vi "IV(H)_DC_vector_magnet_anglesweep_BF_LD-400_K6221_K2182A_PK.vi"() -> ()   [LabVIEW 2016]
uses:
  <vilib>/Math Plots/2D Math Plots/2D Compass/2D Compass XCtrl/2D Compass.xctl
  <vilib>/Math Plots/2D Math Plots/2D Compass/2D Compass Datatype/2D Compass Datatype.lvclass
  <vilib>/Math Plots/2D Math Plots/2D Compass/2D Compass Datatype/Public/Plot Helper (Vector).vi
  Labview Drivers/Keithley 622x LV 2009/Keithley 622x.lvlib
panel:
  out "2D Compass":refnum<class "2D Plot Datatype.lvclass">[](xcontrol)
  in  "Set Compliance voltage (V)":dbl=5.0 min=0.0 step=0.1 format="%_3f"
  in  "Step 3":dbl[](array[numeric])=[2e-06, 0.0001, 2e-06, 1e-06] min=-3000.0 max=3000.0 format="%.3e"
  in  "To 3":dbl[](array[numeric])=[0.00032, 1e-06, -0.00032, -1e-06] min=-3000.0 max=3000.0 format="%.1e"
  in  "From 3":dbl[](array[numeric])=[0.0, 0.00032, 0.0, -0.00032] min=-3000.0 max=3000.0 format="%.1e"
  in  "wait (ms)":u32=50
  in  "Nanovoltmeter 2182a VISA":refnum<visa-resource-name>="GPIB0::7::INSTR"
  in  "Current source K6221 VISA":refnum<visa-resource-name>="GPIB0::13::INSTR"
  in  "Number Averaging":i32=1
  in  "Tab Control":enum32{"Page 1", "Page 2"}(tab)
  out "V vs I":cluster{dbl, "Field Reading":dbl}[](graph)=[{0.0, "Field Reading"=4.40241798e-08}, {2e-08, "Field Reading"=1.23783257e-07}, {4e-08, "Field Reading"=3.02986118e-07}, {6e-08, "Field Reading"=5.49519534e-07}, {8e-08, "Field Reading"=7.0386157e-07}, {1e-07, "Field Reading"=8.50435e-07}, {1.2e-07, "Field Reading"=1.09593255e-06}, {1.4e-07, "Field Reading"=1.21350074e-06}, {1.6e-07, "Field Reading"=1.39529319e-06}, {1.8e-07, "Field Reading"=1.54134866e-06}, {2e-07, "Field Reading"=1.75991058e-06}, {2.2e-07, "Field Reading"=1.91891414e-06}, {2.4e-07, "Field Reading"=2.05875441e-06}, {2.6e-07, "Field Reading"=2.23173979e-06}, {2.8e-07, "Field Reading"=2.36018563e-06}, {3e-07, "Field Reading"=2.64452742e-06}, {3.2e-07, "Field Reading"=2.75122088e-06}, {3.4e-07, "Field Reading"=2.90763477e-06}, {3.6e-07, "Field Reading"=3.12050268e-06}, {3.8e-07, "Field Reading"=3.23392292e-06}, {4e-07, "Field Reading"=3.48200967e-06}, {4.2e-07, "Field Reading"=3.63013662e-06}, {4.4e-07, "Field Reading"=3.79483537e-06}, {4.6e-07, "Field Reading"=3.94296229e-06}, {4.8e-07, "Field Reading"=4.10869871e-06}, {5e-07, "Field Reading"=4.332443e-06}, {5.2e-07, "Field Reading"=4.44638679e-06}, {5.4e-07, "Field Reading"=4.61160528e-06}, {5.6e-07, "Field Reading"=4.8415635e-06}, {5.8e-07, "Field Reading"=4.99228004e-06}, {6e-07, "Field Reading"=5.17562593e-06}, {6.2e-07, "Field Reading"=5.33774246e-06}, {6.4e-07, "Field Reading"=5.53403662e-06}, {6.6e-07, "Field Reading"=5.65315972e-06}, {6.8e-07, "Field Reading"=5.83340484e-06}, {7e-07, "Field Reading"=6.04161144e-06}, {7.2e-07, "Field Reading"=6.14312511e-06}, {7.4e-07, "Field Reading"=6.37827086e-06}, {7.6e-07, "Field Reading"=6.53727451e-06}, {7.8e-07, "Field Reading"=6.69938572e-06}, {8e-07, "Field Reading"=6.88635475e-06}, {8.2e-07, "Field Reading"=7.02101579e-06}, {8.4e-07, "Field Reading"=7.23699138e-06}, {8.6e-07, "Field Reading"=7.41308471e-06}, {8.8e-07, "Field Reading"=7.58244684e-06}, {9e-07, "Field Reading"=7.74041457e-06}, {9.2e-07, "Field Reading"=7.90562381e-06}, {9.4e-07, "Field Reading"=8.06618106e-06}, {9.6e-07, "Field Reading"=8.2422761e-06}, {9.8e-07, "Field Reading"=8.41162272e-06}, {1e-06, "Field Reading"=8.59082511e-06}, {1.02e-06, "Field Reading"=8.73842623e-06}, {1.04e-06, "Field Reading"=8.94248895e-06}, {1.06e-06, "Field Reading"=9.14240827e-06}, {1.08e-06, "Field Reading"=9.27862314e-06}, {1.1e-06, "Field Reading"=9.47388113e-06}, {1.12e-06, "Field Reading"=9.62770506e-06}, {1.14e-06, "Field Reading"=9.81261485e-06}, {1.16e-06, "Field Reading"=9.94365015e-06}, {1.18e-06, "Field Reading"=1.0168948e-05}, {1.2e-06, "Field Reading"=1.03238199e-05}, {1.22e-06, "Field Reading"=1.05263292e-05}, {1.24e-06, "Field Reading"=1.0654257e-05}, {1.26e-06, "Field Reading"=1.08365675e-05}, {1.28e-06, "Field Reading"=1.09608698e-05}, {1.3e-06, "Field Reading"=1.11291959e-05}, {1.32e-06, "Field Reading"=1.13104759e-05}, {1.34e-06, "Field Reading"=1.14658539e-05}, {1.36e-06, "Field Reading"=1.17056539e-05}, {1.38e-06, "Field Reading"=1.1880715e-05}, {1.4e-06, "Field Reading"=1.20252166e-05}, {1.42e-06, "Field Reading"=1.22121882e-05}, {1.44e-06, "Field Reading"=1.23541037e-05}, {1.46e-06, "Field Reading"=1.2493426e-05}, {1.48e-06, "Field Reading"=1.27368517e-05}, {1.5e-06, "Field Reading"=1.28668613e-05}, {1.52e-06, "Field Reading"=1.3010845e-05}, {1.54e-06, "Field Reading"=1.31729562e-05}, {1.56e-06, "Field Reading"=1.34153398e-05}, {1.58e-06, "Field Reading"=1.3541714e-05}, {1.6e-06, "Field Reading"=1.36877694e-05}, {1.62e-06, "Field Reading"=1.38659327e-05}, {1.64e-06, "Field Reading"=1.40705138e-05}, {1.66e-06, "Field Reading"=1.42554137e-05}, {1.68e-06, "Field Reading"=1.43978348e-05}, {1.7e-06, "Field Reading"=1.45537307e-05}, {1.72e-06, "Field Reading"=1.4763491e-05}, {1.74e-06, "Field Reading"=1.49478731e-05}, {1.76e-06, "Field Reading"=1.50571556e-05}, {1.78e-06, "Field Reading"=1.5244645e-05}, {1.8e-06, "Field Reading"=1.54171202e-05}, {1.82e-06, "Field Reading"=1.55590321e-05}, {1.84e-06, "Field Reading"=1.57708642e-05}, {1.86e-06, "Field Reading"=1.59593796e-05}, {1.88e-06, "Field Reading"=1.60826461e-05}, {1.9e-06, "Field Reading"=1.62836016e-05}, {1.92e-06, "Field Reading"=1.64534904e-05}, {1.94e-06, "Field Reading"=1.65871155e-05}, {1.96e-06, "Field Reading"=1.68072344e-05}, {1.98e-06, "Field Reading"=1.69807332e-05}, {2e-06, "Field Reading"=1.71039997e-05}, {2.02e-06, "Field Reading"=1.73298157e-05}, {2.04e-06, "Field Reading"=1.75338777e-05}, {2.06e-06, "Field Reading"=1.76706104e-05}, {2.08e-06, "Field Reading"=1.78063071e-05}, {2.1e-06, "Field Reading"=1.79881126e-05}, {2.12e-06, "Field Reading"=1.81730125e-05}, {2.14e-06, "Field Reading"=1.83542869e-05}, {2.16e-06, "Field Reading"=1.84765118e-05}, {2.18e-06, "Field Reading"=1.86950769e-05}, {2.2e-06, "Field Reading"=1.88804946e-05}, {2.22e-06, "Field Reading"=1.90384784e-05}, {2.24e-06, "Field Reading"=1.91767649e-05}, {2.26e-06, "Field Reading"=1.93580394e-05}, {2.28e-06, "Field Reading"=1.95553725e-05}, {2.3e-06, "Field Reading"=1.97330215e-05}, {2.32e-06, "Field Reading"=1.98827024e-05}, {2.34e-06, "Field Reading"=2.00670785e-05}, {2.36e-06, "Field Reading"=2.02561219e-05}, {2.38e-06, "Field Reading"=2.04550059e-05}, {2.4e-06, "Field Reading"=2.05839566e-05}, {2.42e-06, "Field Reading"=2.07004901e-05}, {2.44e-06, "Field Reading"=2.08941947e-05}, {2.46e-06, "Field Reading"=2.10935914e-05}, {2.48e-06, "Field Reading"=2.12541486e-05}, {2.5e-06, "Field Reading"=2.14209052e-05}, {2.52e-06, "Field Reading"=2.16146097e-05}, {2.54e-06, "Field Reading"=2.18026169e-05}, {2.56e-06, "Field Reading"=2.19916641e-05}, {2.58e-06, "Field Reading"=2.21568827e-05}, {2.6e-06, "Field Reading"=2.23319418e-05}, {2.62e-06, "Field Reading"=2.2459882e-05}, {2.64e-06, "Field Reading"=2.26406384e-05}, {2.66e-06, "Field Reading"=2.28395223e-05}, {2.68e-06, "Field Reading"=2.2994903e-05}, {2.7e-06, "Field Reading"=2.31471734e-05}, {2.72e-06, "Field Reading"=2.32978901e-05}, {2.74e-06, "Field Reading"=2.34921259e-05}, {2.76e-06, "Field Reading"=2.36547549e-05}, {2.78e-06, "Field Reading"=2.38215274e-05}, {2.8e-06, "Field Reading"=2.40152458e-05}, {2.82e-06, "Field Reading"=2.41934127e-05}, {2.84e-06, "Field Reading"=2.43938505e-05}, {2.86e-06, "Field Reading"=2.4514533e-05}, {2.88e-06, "Field Reading"=2.47548513e-05}, {2.9e-06, "Field Reading"=2.48532575e-05}, {2.92e-06, "Field Reading"=2.50619679e-05}, {2.94e-06, "Field Reading"=2.51930034e-05}, {2.96e-06, "Field Reading"=2.5380493e-05}, {2.98e-06, "Field Reading"=2.55322419e-05}, {3e-06, "Field Reading"=2.57492533e-05}, {3e-06, "Field Reading"=2.57720421e-05}, {2e-06, "Field Reading"=1.71412944e-05}, {1e-06, "Field Reading"=8.50279535e-06}, {0.0, "Field Reading"=-1.17576765e-07}, {-2e-08, "Field Reading"=-2.68811351e-07}, {-4e-08, "Field Reading"=-4.69766897e-07}, {-6e-08, "Field Reading"=-6.21518846e-07}, {-8e-08, "Field Reading"=-8.17295154e-07}, {-1e-07, "Field Reading"=-9.41079645e-07}, {-1.2e-07, "Field Reading"=-1.18502315e-06}, {-1.4e-07, "Field Reading"=-1.34454459e-06}, {-1.6e-07, "Field Reading"=-1.46573945e-06}, {-1.8e-07, "Field Reading"=-1.69051911e-06}, {-2e-07, "Field Reading"=-1.82621594e-06}, {-2.2e-07, "Field Reading"=-2.0126696e-06}, {-2.4e-07, "Field Reading"=-2.21776914e-06}, {-2.6e-07, "Field Reading"=-2.35450179e-06}, {-2.8e-07, "Field Reading"=-2.58601504e-06}, {-3e-07, "Field Reading"=-2.69322674e-06}, {-3.2e-07, "Field Reading"=-2.83721031e-06}, {-3.4e-07, "Field Reading"=-3.08995843e-06}, {-3.6e-07, "Field Reading"=-3.19457944e-06}, {-3.8e-07, "Field Reading"=-3.37844337e-06}, {-4e-07, "Field Reading"=-3.57266625e-06}, {-4.2e-07, "Field Reading"=-3.76792448e-06}, {-4.4e-07, "Field Reading"=-3.93469675e-06}, {-4.6e-07, "Field Reading"=-4.04864062e-06}, {-4.8e-07, "Field Reading"=-4.20505435e-06}, {-5e-07, "Field Reading"=-4.46867881e-06}, {-5.2e-07, "Field Reading"=-4.63596869e-06}, {-5.4e-07, "Field Reading"=-4.79238132e-06}, {-5.6e-07, "Field Reading"=-4.99799659e-06}, {-5.8e-07, "Field Reading"=-5.13783554e-06}, {-6e-07, "Field Reading"=-5.31133956e-06}, {-6.2e-07, "Field Reading"=-5.45014278e-06}, {-6.4e-07, "Field Reading"=-5.69460221e-06}, {-6.6e-07, "Field Reading"=-5.77436228e-06}, {-6.8e-07, "Field Reading"=-5.97428035e-06}, {-7e-07, "Field Reading"=-6.12913905e-06}, {-7.2e-07, "Field Reading"=-6.38136727e-06}, {-7.4e-07, "Field Reading"=-6.52534971e-06}, {-7.6e-07, "Field Reading"=-6.63359599e-06}, {-7.8e-07, "Field Reading"=-6.85112346e-06}, {-8e-07, "Field Reading"=-7.07020515e-06}, {-8.2e-07, "Field Reading"=-7.20641881e-06}, {-8.4e-07, "Field Reading"=-7.40167564e-06}, {-8.6e-07, "Field Reading"=-7.54669386e-06}, {-8.8e-07, "Field Reading"=-7.71035741e-06}, {-9e-07, "Field Reading"=-7.89525579e-06}, {-9.2e-07, "Field Reading"=-8.04286623e-06}, {-9.4e-07, "Field Reading"=-8.20031482e-06}, {-9.6e-07, "Field Reading"=-8.37226526e-06}, {-9.8e-07, "Field Reading"=-8.56441587e-06}, {-1e-06, "Field Reading"=-8.75760121e-06}, {-1.02e-06, "Field Reading"=-8.97305724e-06}, {-1.04e-06, "Field Reading"=-9.09994792e-06}, {-1.06e-06, "Field Reading"=-9.267755e-06}, {-1.08e-06, "Field Reading"=-9.48372893e-06}, {-1.1e-06, "Field Reading"=-9.64739249e-06}, {-1.12e-06, "Field Reading"=-9.79396472e-06}, {-1.14e-06, "Field Reading"=-9.97938118e-06}, {-1.16e-06, "Field Reading"=-1.00990192e-05}, {-1.18e-06, "Field Reading"=-1.03647137e-05}, {-1.2e-06, "Field Reading"=-1.04952302e-05}, {-1.22e-06, "Field Reading"=-1.06247112e-05}, {-1.24e-06, "Field Reading"=-1.08479359e-05}, {-1.26e-06, "Field Reading"=-1.10452646e-05}, {-1.28e-06, "Field Reading"=-1.11291712e-05}, {-1.3e-06, "Field Reading"=-1.13979733e-05}, {-1.32e-06, "Field Reading"=-1.15290079e-05}, {-1.34e-06, "Field Reading"=-1.17107996e-05}, {-1.36e-06, "Field Reading"=-1.18584077e-05}, {-1.38e-06, "Field Reading"=-1.2031394e-05}, {-1.4e-06, "Field Reading"=-1.22214705e-05}, {-1.42e-06, "Field Reading"=-1.23742578e-05}, {-1.44e-06, "Field Reading"=-1.25384394e-05}, {-1.46e-06, "Field Reading"=-1.27621798e-05}, {-1.48e-06, "Field Reading"=-1.28792304e-05}, {-1.5e-06, "Field Reading"=-1.30289101e-05}, {-1.52e-06, "Field Reading"=-1.32428105e-05}, {-1.54e-06, "Field Reading"=-1.34660352e-05}, {-1.56e-06, "Field Reading"=-1.35644406e-05}, {-1.58e-06, "Field Reading"=-1.37255157e-05}, {-1.6e-06, "Field Reading"=-1.39409717e-05}, {-1.62e-06, "Field Reading"=-1.41439974e-05}, {-1.64e-06, "Field Reading"=-1.42952297e-05}, {-1.66e-06, "Field Reading"=-1.44941121e-05}, {-1.68e-06, "Field Reading"=-1.45919995e-05}, {-1.7e-06, "Field Reading"=-1.47965808e-05}, {-1.72e-06, "Field Reading"=-1.50275744e-05}, {-1.74e-06, "Field Reading"=-1.51088883e-05}, {-1.76e-06, "Field Reading"=-1.5286534e-05}, {-1.78e-06, "Field Reading"=-1.55475671e-05}, {-1.8e-06, "Field Reading"=-1.56418291e-05}, {-1.82e-06, "Field Reading"=-1.58401957e-05}, {-1.84e-06, "Field Reading"=-1.60354527e-05}, {-1.86e-06, "Field Reading"=-1.61778815e-05}, {-1.88e-06, "Field Reading"=-1.64109433e-05}, {-1.9e-06, "Field Reading"=-1.65114203e-05}, {-1.92e-06, "Field Reading"=-1.67460393e-05}, {-1.94e-06, "Field Reading"=-1.69164354e-05}, {-1.96e-06, "Field Reading"=-1.7107031e-05}, {-1.98e-06, "Field Reading"=-1.72157948e-05}, {-2e-06, "Field Reading"=-1.73789424e-05}, {-2.02e-06, "Field Reading"=-1.7616151e-05}, {-2.04e-06, "Field Reading"=-1.77135205e-05}, {-2.06e-06, "Field Reading"=-1.788599e-05}, {-2.08e-06, "Field Reading"=-1.80781394e-05}, {-2.1e-06, "Field Reading"=-1.82045126e-05}, {-2.12e-06, "Field Reading"=-1.84603712e-05}, {-2.14e-06, "Field Reading"=-1.8589852e-05}, {-2.16e-06, "Field Reading"=-1.87690534e-05}, {-2.18e-06, "Field Reading"=-1.89917572e-05}, {-2.2e-06, "Field Reading"=-1.91388473e-05}, {-2.22e-06, "Field Reading"=-1.93584466e-05}, {-2.24e-06, "Field Reading"=-1.95366097e-05}, {-2.26e-06, "Field Reading"=-1.96655725e-05}, {-2.28e-06, "Field Reading"=-1.98468455e-05}, {-2.3e-06, "Field Reading"=-2.00260392e-05}, {-2.32e-06, "Field Reading"=-2.02104196e-05}, {-2.34e-06, "Field Reading"=-2.03642427e-05}, {-2.36e-06, "Field Reading"=-2.05486354e-05}, {-2.38e-06, "Field Reading"=-2.07009048e-05}, {-2.4e-06, "Field Reading"=-2.08485128e-05}, {-2.42e-06, "Field Reading"=-2.10551707e-05}, {-2.44e-06, "Field Reading"=-2.12468023e-05}, {-2.46e-06, "Field Reading"=-2.14161632e-05}, {-2.48e-06, "Field Reading"=-2.1574128e-05}, {-2.5e-06, "Field Reading"=-2.17181107e-05}, {-2.52e-06, "Field Reading"=-2.18755593e-05}, {-2.54e-06, "Field Reading"=-2.21179489e-05}, {-2.56e-06, "Field Reading"=-2.22878278e-05}, {-2.58e-06, "Field Reading"=-2.246185e-05}, {-2.6e-06, "Field Reading"=-2.26146323e-05}, {-2.62e-06, "Field Reading"=-2.28161044e-05}, {-2.64e-06, "Field Reading"=-2.29424776e-05}, {-2.66e-06, "Field Reading"=-2.30880191e-05}, {-2.68e-06, "Field Reading"=-2.32863837e-05}, {-2.7e-06, "Field Reading"=-2.34681748e-05}, {-2.72e-06, "Field Reading"=-2.36484132e-05}, {-2.74e-06, "Field Reading"=-2.38566183e-05}, {-2.76e-06, "Field Reading"=-2.39985293e-05}, {-2.78e-06, "Field Reading"=-2.41513117e-05}, {-2.8e-06, "Field Reading"=-2.43227442e-05}, {-2.82e-06, "Field Reading"=-2.44646552e-05}, {-2.84e-06, "Field Reading"=-2.46112313e-05}, {-2.86e-06, "Field Reading"=-2.47919865e-05}, {-2.88e-06, "Field Reading"=-2.50271236e-05}, {-2.9e-06, "Field Reading"=-2.51327718e-05}, {-2.92e-06, "Field Reading"=-2.53295825e-05}, {-2.94e-06, "Field Reading"=-2.55269109e-05}, {-2.96e-06, "Field Reading"=-2.57024868e-05}, {-2.98e-06, "Field Reading"=-2.5883242e-05}, {-3e-06, "Field Reading"=-2.59930485e-05}, {-3e-06, "Field Reading"=-2.60981869e-05}, {-2e-06, "Field Reading"=-1.74783916e-05}]
  out "V vs time":cluster{dbl, "Field Reading":dbl}[](graph)=[{14037.38, "Field Reading"=4.40241798e-08}, {14037.632, "Field Reading"=1.23783257e-07}, {14037.885, "Field Reading"=3.02986118e-07}, {14038.144, "Field Reading"=5.49519534e-07}, {14038.396, "Field Reading"=7.0386157e-07}, {14038.649, "Field Reading"=8.50435e-07}, {14038.901, "Field Reading"=1.09593255e-06}, {14039.16, "Field Reading"=1.21350074e-06}, {14039.412, "Field Reading"=1.39529319e-06}, {14039.666, "Field Reading"=1.54134866e-06}, {14039.921, "Field Reading"=1.75991058e-06}, {14040.178, "Field Reading"=1.91891414e-06}, {14040.432, "Field Reading"=2.05875441e-06}, {14040.684, "Field Reading"=2.23173979e-06}, {14040.944, "Field Reading"=2.36018563e-06}, {14041.201, "Field Reading"=2.64452742e-06}, {14041.453, "Field Reading"=2.75122088e-06}, {14041.705, "Field Reading"=2.90763477e-06}, {14041.964, "Field Reading"=3.12050268e-06}, {14042.218, "Field Reading"=3.23392292e-06}, {14042.47, "Field Reading"=3.48200967e-06}, {14042.726, "Field Reading"=3.63013662e-06}, {14042.982, "Field Reading"=3.79483537e-06}, {14043.242, "Field Reading"=3.94296229e-06}, {14043.495, "Field Reading"=4.10869871e-06}, {14043.747, "Field Reading"=4.332443e-06}, {14043.999, "Field Reading"=4.44638679e-06}, {14044.252, "Field Reading"=4.61160528e-06}, {14044.507, "Field Reading"=4.8415635e-06}, {14044.761, "Field Reading"=4.99228004e-06}, {14045.019, "Field Reading"=5.17562593e-06}, {14045.274, "Field Reading"=5.33774246e-06}, {14045.526, "Field Reading"=5.53403662e-06}, {14045.778, "Field Reading"=5.65315972e-06}, {14046.028, "Field Reading"=5.83340484e-06}, {14046.282, "Field Reading"=6.04161144e-06}, {14046.538, "Field Reading"=6.14312511e-06}, {14046.794, "Field Reading"=6.37827086e-06}, {14047.048, "Field Reading"=6.53727451e-06}, {14047.299, "Field Reading"=6.69938572e-06}, {14047.553, "Field Reading"=6.88635475e-06}, {14047.806, "Field Reading"=7.02101579e-06}, {14048.061, "Field Reading"=7.23699138e-06}, {14048.315, "Field Reading"=7.41308471e-06}, {14048.572, "Field Reading"=7.58244684e-06}, {14048.825, "Field Reading"=7.74041457e-06}, {14049.076, "Field Reading"=7.90562381e-06}, {14049.332, "Field Reading"=8.06618106e-06}, {14049.585, "Field Reading"=8.2422761e-06}, {14049.845, "Field Reading"=8.41162272e-06}, {14050.098, "Field Reading"=8.59082511e-06}, {14050.354, "Field Reading"=8.73842623e-06}, {14050.61, "Field Reading"=8.94248895e-06}, {14050.867, "Field Reading"=9.14240827e-06}, {14051.121, "Field Reading"=9.27862314e-06}, {14051.375, "Field Reading"=9.47388113e-06}, {14051.632, "Field Reading"=9.62770506e-06}, {14051.888, "Field Reading"=9.81261485e-06}, {14052.138, "Field Reading"=9.94365015e-06}, {14052.392, "Field Reading"=1.0168948e-05}, {14052.645, "Field Reading"=1.03238199e-05}, {14052.897, "Field Reading"=1.05263292e-05}, {14053.15, "Field Reading"=1.0654257e-05}, {14053.405, "Field Reading"=1.08365675e-05}, {14053.659, "Field Reading"=1.09608698e-05}, {14053.913, "Field Reading"=1.11291959e-05}, {14054.167, "Field Reading"=1.13104759e-05}, {14054.419, "Field Reading"=1.14658539e-05}, {14054.67, "Field Reading"=1.17056539e-05}, {14054.922, "Field Reading"=1.1880715e-05}, {14055.177, "Field Reading"=1.20252166e-05}, {14055.434, "Field Reading"=1.22121882e-05}, {14055.689, "Field Reading"=1.23541037e-05}, {14055.94, "Field Reading"=1.2493426e-05}, {14056.191, "Field Reading"=1.27368517e-05}, {14056.449, "Field Reading"=1.28668613e-05}, {14056.699, "Field Reading"=1.3010845e-05}, {14056.952, "Field Reading"=1.31729562e-05}, {14057.208, "Field Reading"=1.34153398e-05}, {14057.46, "Field Reading"=1.3541714e-05}, {14057.716, "Field Reading"=1.36877694e-05}, {14057.967, "Field Reading"=1.38659327e-05}, {14058.221, "Field Reading"=1.40705138e-05}, {14058.476, "Field Reading"=1.42554137e-05}, {14058.73, "Field Reading"=1.43978348e-05}, {14058.981, "Field Reading"=1.45537307e-05}, {14059.24, "Field Reading"=1.4763491e-05}, {14059.494, "Field Reading"=1.49478731e-05}, {14059.745, "Field Reading"=1.50571556e-05}, {14059.996, "Field Reading"=1.5244645e-05}, {14060.254, "Field Reading"=1.54171202e-05}, {14060.516, "Field Reading"=1.55590321e-05}, {14060.772, "Field Reading"=1.57708642e-05}, {14061.025, "Field Reading"=1.59593796e-05}, {14061.279, "Field Reading"=1.60826461e-05}, {14061.53, "Field Reading"=1.62836016e-05}, {14061.784, "Field Reading"=1.64534904e-05}, {14062.036, "Field Reading"=1.65871155e-05}, {14062.29, "Field Reading"=1.68072344e-05}, {14062.54, "Field Reading"=1.69807332e-05}, {14062.796, "Field Reading"=1.71039997e-05}, {14063.053, "Field Reading"=1.73298157e-05}, {14063.309, "Field Reading"=1.75338777e-05}, {14063.566, "Field Reading"=1.76706104e-05}, {14063.826, "Field Reading"=1.78063071e-05}, {14064.081, "Field Reading"=1.79881126e-05}, {14064.335, "Field Reading"=1.81730125e-05}, {14064.589, "Field Reading"=1.83542869e-05}, {14064.843, "Field Reading"=1.84765118e-05}, {14065.098, "Field Reading"=1.86950769e-05}, {14065.349, "Field Reading"=1.88804946e-05}, {14065.606, "Field Reading"=1.90384784e-05}, {14065.856, "Field Reading"=1.91767649e-05}, {14066.114, "Field Reading"=1.93580394e-05}, {14066.37, "Field Reading"=1.95553725e-05}, {14066.623, "Field Reading"=1.97330215e-05}, {14066.877, "Field Reading"=1.98827024e-05}, {14067.132, "Field Reading"=2.00670785e-05}, {14067.38, "Field Reading"=2.02561219e-05}, {14067.639, "Field Reading"=2.04550059e-05}, {14067.895, "Field Reading"=2.05839566e-05}, {14068.147, "Field Reading"=2.07004901e-05}, {14068.401, "Field Reading"=2.08941947e-05}, {14068.659, "Field Reading"=2.10935914e-05}, {14068.911, "Field Reading"=2.12541486e-05}, {14069.172, "Field Reading"=2.14209052e-05}, {14069.43, "Field Reading"=2.16146097e-05}, {14069.684, "Field Reading"=2.18026169e-05}, {14069.94, "Field Reading"=2.19916641e-05}, {14070.193, "Field Reading"=2.21568827e-05}, {14070.445, "Field Reading"=2.23319418e-05}, {14070.699, "Field Reading"=2.2459882e-05}, {14070.952, "Field Reading"=2.26406384e-05}, {14071.245, "Field Reading"=2.28395223e-05}, {14071.499, "Field Reading"=2.2994903e-05}, {14071.751, "Field Reading"=2.31471734e-05}, {14072.002, "Field Reading"=2.32978901e-05}, {14072.256, "Field Reading"=2.34921259e-05}, {14072.514, "Field Reading"=2.36547549e-05}, {14072.771, "Field Reading"=2.38215274e-05}, {14073.029, "Field Reading"=2.40152458e-05}, {14073.283, "Field Reading"=2.41934127e-05}, {14073.538, "Field Reading"=2.43938505e-05}, {14073.795, "Field Reading"=2.4514533e-05}, {14074.05, "Field Reading"=2.47548513e-05}, {14074.304, "Field Reading"=2.48532575e-05}, {14074.561, "Field Reading"=2.50619679e-05}, {14074.816, "Field Reading"=2.51930034e-05}, {14075.073, "Field Reading"=2.5380493e-05}, {14075.33, "Field Reading"=2.55322419e-05}, {14075.586, "Field Reading"=2.57492533e-05}, {14075.839, "Field Reading"=2.57720421e-05}, {14076.092, "Field Reading"=1.71412944e-05}, {14076.348, "Field Reading"=8.50279535e-06}, {14076.604, "Field Reading"=-1.17576765e-07}, {14076.861, "Field Reading"=-2.68811351e-07}, {14077.119, "Field Reading"=-4.69766897e-07}, {14077.374, "Field Reading"=-6.21518846e-07}, {14077.629, "Field Reading"=-8.17295154e-07}, {14077.885, "Field Reading"=-9.41079645e-07}, {14078.14, "Field Reading"=-1.18502315e-06}, {14078.396, "Field Reading"=-1.34454459e-06}, {14078.651, "Field Reading"=-1.46573945e-06}, {14078.907, "Field Reading"=-1.69051911e-06}, {14079.159, "Field Reading"=-1.82621594e-06}, {14079.411, "Field Reading"=-2.0126696e-06}, {14079.666, "Field Reading"=-2.21776914e-06}, {14079.921, "Field Reading"=-2.35450179e-06}, {14080.176, "Field Reading"=-2.58601504e-06}, {14080.431, "Field Reading"=-2.69322674e-06}, {14080.686, "Field Reading"=-2.83721031e-06}, {14080.941, "Field Reading"=-3.08995843e-06}, {14081.197, "Field Reading"=-3.19457944e-06}, {14081.456, "Field Reading"=-3.37844337e-06}, {14081.712, "Field Reading"=-3.57266625e-06}, {14081.965, "Field Reading"=-3.76792448e-06}, {14082.226, "Field Reading"=-3.93469675e-06}, {14082.488, "Field Reading"=-4.04864062e-06}, {14082.744, "Field Reading"=-4.20505435e-06}, {14082.996, "Field Reading"=-4.46867881e-06}, {14083.251, "Field Reading"=-4.63596869e-06}, {14083.511, "Field Reading"=-4.79238132e-06}, {14083.765, "Field Reading"=-4.99799659e-06}, {14084.021, "Field Reading"=-5.13783554e-06}, {14084.276, "Field Reading"=-5.31133956e-06}, {14084.527, "Field Reading"=-5.45014278e-06}, {14084.782, "Field Reading"=-5.69460221e-06}, {14085.035, "Field Reading"=-5.77436228e-06}, {14085.291, "Field Reading"=-5.97428035e-06}, {14085.549, "Field Reading"=-6.12913905e-06}, {14085.804, "Field Reading"=-6.38136727e-06}, {14086.059, "Field Reading"=-6.52534971e-06}, {14086.312, "Field Reading"=-6.63359599e-06}, {14086.57, "Field Reading"=-6.85112346e-06}, {14086.856, "Field Reading"=-7.07020515e-06}, {14087.114, "Field Reading"=-7.20641881e-06}, {14087.366, "Field Reading"=-7.40167564e-06}, {14087.614, "Field Reading"=-7.54669386e-06}, {14087.867, "Field Reading"=-7.71035741e-06}, {14088.116, "Field Reading"=-7.89525579e-06}, {14088.367, "Field Reading"=-8.04286623e-06}, {14088.619, "Field Reading"=-8.20031482e-06}, {14088.873, "Field Reading"=-8.37226526e-06}, {14089.129, "Field Reading"=-8.56441587e-06}, {14089.384, "Field Reading"=-8.75760121e-06}, {14089.636, "Field Reading"=-8.97305724e-06}, {14089.892, "Field Reading"=-9.09994792e-06}, {14090.149, "Field Reading"=-9.267755e-06}, {14090.401, "Field Reading"=-9.48372893e-06}, {14090.657, "Field Reading"=-9.64739249e-06}, {14090.907, "Field Reading"=-9.79396472e-06}, {14091.159, "Field Reading"=-9.97938118e-06}, {14091.416, "Field Reading"=-1.00990192e-05}, {14091.665, "Field Reading"=-1.03647137e-05}, {14091.915, "Field Reading"=-1.04952302e-05}, {14092.167, "Field Reading"=-1.06247112e-05}, {14092.423, "Field Reading"=-1.08479359e-05}, {14092.677, "Field Reading"=-1.10452646e-05}, {14092.929, "Field Reading"=-1.11291712e-05}, {14093.18, "Field Reading"=-1.13979733e-05}, {14093.431, "Field Reading"=-1.15290079e-05}, {14093.686, "Field Reading"=-1.17107996e-05}, {14093.939, "Field Reading"=-1.18584077e-05}, {14094.193, "Field Reading"=-1.2031394e-05}, {14094.445, "Field Reading"=-1.22214705e-05}, {14094.697, "Field Reading"=-1.23742578e-05}, {14094.948, "Field Reading"=-1.25384394e-05}, {14095.202, "Field Reading"=-1.27621798e-05}, {14095.455, "Field Reading"=-1.28792304e-05}, {14095.706, "Field Reading"=-1.30289101e-05}, {14095.961, "Field Reading"=-1.32428105e-05}, {14096.213, "Field Reading"=-1.34660352e-05}, {14096.47, "Field Reading"=-1.35644406e-05}, {14096.723, "Field Reading"=-1.37255157e-05}, {14096.973, "Field Reading"=-1.39409717e-05}, {14097.227, "Field Reading"=-1.41439974e-05}, {14097.479, "Field Reading"=-1.42952297e-05}, {14097.732, "Field Reading"=-1.44941121e-05}, {14097.986, "Field Reading"=-1.45919995e-05}, {14098.24, "Field Reading"=-1.47965808e-05}, {14098.495, "Field Reading"=-1.50275744e-05}, {14098.749, "Field Reading"=-1.51088883e-05}, {14099.002, "Field Reading"=-1.5286534e-05}, {14099.255, "Field Reading"=-1.55475671e-05}, {14099.512, "Field Reading"=-1.56418291e-05}, {14099.766, "Field Reading"=-1.58401957e-05}, {14100.016, "Field Reading"=-1.60354527e-05}, {14100.266, "Field Reading"=-1.61778815e-05}, {14100.518, "Field Reading"=-1.64109433e-05}, {14100.77, "Field Reading"=-1.65114203e-05}, {14101.021, "Field Reading"=-1.67460393e-05}, {14101.275, "Field Reading"=-1.69164354e-05}, {14101.528, "Field Reading"=-1.7107031e-05}, {14101.783, "Field Reading"=-1.72157948e-05}, {14102.039, "Field Reading"=-1.73789424e-05}, {14102.294, "Field Reading"=-1.7616151e-05}, {14102.546, "Field Reading"=-1.77135205e-05}, {14102.796, "Field Reading"=-1.788599e-05}, {14103.051, "Field Reading"=-1.80781394e-05}, {14103.303, "Field Reading"=-1.82045126e-05}, {14103.556, "Field Reading"=-1.84603712e-05}, {14103.81, "Field Reading"=-1.8589852e-05}, {14104.061, "Field Reading"=-1.87690534e-05}, {14104.316, "Field Reading"=-1.89917572e-05}, {14104.567, "Field Reading"=-1.91388473e-05}, {14104.819, "Field Reading"=-1.93584466e-05}, {14105.072, "Field Reading"=-1.95366097e-05}, {14105.328, "Field Reading"=-1.96655725e-05}, {14105.579, "Field Reading"=-1.98468455e-05}, {14105.838, "Field Reading"=-2.00260392e-05}, {14106.091, "Field Reading"=-2.02104196e-05}, {14106.341, "Field Reading"=-2.03642427e-05}, {14106.595, "Field Reading"=-2.05486354e-05}, {14106.848, "Field Reading"=-2.07009048e-05}, {14107.103, "Field Reading"=-2.08485128e-05}, {14107.357, "Field Reading"=-2.10551707e-05}, {14107.61, "Field Reading"=-2.12468023e-05}, {14107.863, "Field Reading"=-2.14161632e-05}, {14108.114, "Field Reading"=-2.1574128e-05}, {14108.368, "Field Reading"=-2.17181107e-05}, {14108.62, "Field Reading"=-2.18755593e-05}, {14108.872, "Field Reading"=-2.21179489e-05}, {14109.126, "Field Reading"=-2.22878278e-05}, {14109.379, "Field Reading"=-2.246185e-05}, {14109.636, "Field Reading"=-2.26146323e-05}, {14109.892, "Field Reading"=-2.28161044e-05}, {14110.145, "Field Reading"=-2.29424776e-05}, {14110.396, "Field Reading"=-2.30880191e-05}, {14110.65, "Field Reading"=-2.32863837e-05}, {14110.899, "Field Reading"=-2.34681748e-05}, {14111.151, "Field Reading"=-2.36484132e-05}, {14111.408, "Field Reading"=-2.38566183e-05}, {14111.663, "Field Reading"=-2.39985293e-05}, {14111.914, "Field Reading"=-2.41513117e-05}, {14112.171, "Field Reading"=-2.43227442e-05}, {14112.429, "Field Reading"=-2.44646552e-05}, {14112.682, "Field Reading"=-2.46112313e-05}, {14112.937, "Field Reading"=-2.47919865e-05}, {14113.19, "Field Reading"=-2.50271236e-05}, {14113.442, "Field Reading"=-2.51327718e-05}, {14113.698, "Field Reading"=-2.53295825e-05}, {14113.955, "Field Reading"=-2.55269109e-05}, {14114.211, "Field Reading"=-2.57024868e-05}, {14114.464, "Field Reading"=-2.5883242e-05}, {14114.717, "Field Reading"=-2.59930485e-05}, {14114.973, "Field Reading"=-2.60981869e-05}, {14115.23, "Field Reading"=-1.74783916e-05}]
  out "Magnetic Field Vector Angle":dbl=330.0003030452058 format="%#_13g"
  out "Magnetic Field Vector magnitude (T)":dbl=0.5999981386233562 format="%#_13g"
  in  "From 2":dbl[](array[numeric])=[-0.6] min=-3000.0 max=3000.0 format="%#.5f"
  in  "To 2":dbl[](array[numeric])=[0.6] min=-3000.0 max=3000.0 format="%#.5g"
  in  "Step 2":dbl[](array[numeric])=[0.005] min=-3000.0 max=3000.0 format="%.5e"
  in  "Wait time after each sweep(min)":dbl=0.1 format="%#_13g"
  out "Z-axis Magnetic Field (T)":string="-0.299996321\r\n"
  in  "Y-axis Field ramp rate (T/min)":string="0.025"
  in  "Z-axis Field ramp rate (T/min)":string="0.025"
  out "Z-axis (90 deg)":dbl(slide)=-0.299996321 scale=0.0..3.0
  out "Y-Axis (0deg)":dbl(slide)=0.519615217 scale=0.0..3.0
  out "Y-axis Magnetic Field (T)":string="0.519615217\r\n"
  in  "Magnet IP Address Z-axis":string="169.254.76.2"
  in  "Magnet IP Address Y-axis":string="169.254.212.23"
  out "Resistance (ohm)":dbl=8.739195800000001 format="%#_13g"
  out "Time (s)":dbl=14115.488 format="%#_13g"
  in  "Magnetic field stabilization time (s)":dbl=1.0 format="%#_13g"
  in  "Step":dbl[](array[numeric])=[1.0] min=-3000.0 max=3000.0 format="%.4g"
  in  "To":dbl[](array[numeric])=[146.37] min=-3000.0 max=3000.0 format="%.4f"
  in  "From":dbl[](array[numeric])=[146.37] min=-3000.0 max=3000.0 format="%.4f"
  out "Iset (A)":dbl=-2e-06
  out "Vmeas (V)":dbl=-1.74783916e-05
  in  "Folder":path=path "D:/Pranava/Data/PtTe2/29-10-2022/002"
  out "data":dbl[](array[numeric])=[0.5999981386233562, 330.0003030452058, -2e-06, -1.74783916e-05, 8.739195800000001, 14115.23]
  in  "File name":string="027_29-10-2022_002_DevH3_I_46-48_V_45-43_DC_IV(H)_baseT_[-600mT_to_600mT]_IP_[146deg]_5mT_steps"
  out "File path":path=path "D:/Pranava/Data/PtTe2/29-10-2022/002/025_29-10-2022_002_DevD2_I_39-36_V_42-41_DC_IV(H)_baseT_[450mT_to_-650mT]_IP_[150deg]_10mT_steps.dat"
  # "Z-Axis: In-plane (90 deg)\nY-axis: Out-of-plane (0 deg)"
  # "[Must be less than 0.05]"
  # ".dat"
  # "It is important that there is enough time for the magnet to cool down after each sweep (Typically 15-20 min)"
  # "Configure Field magnitude (T)"
  # "Configure Field Angle (deg)"
  # "Configure current sweeps (A)"
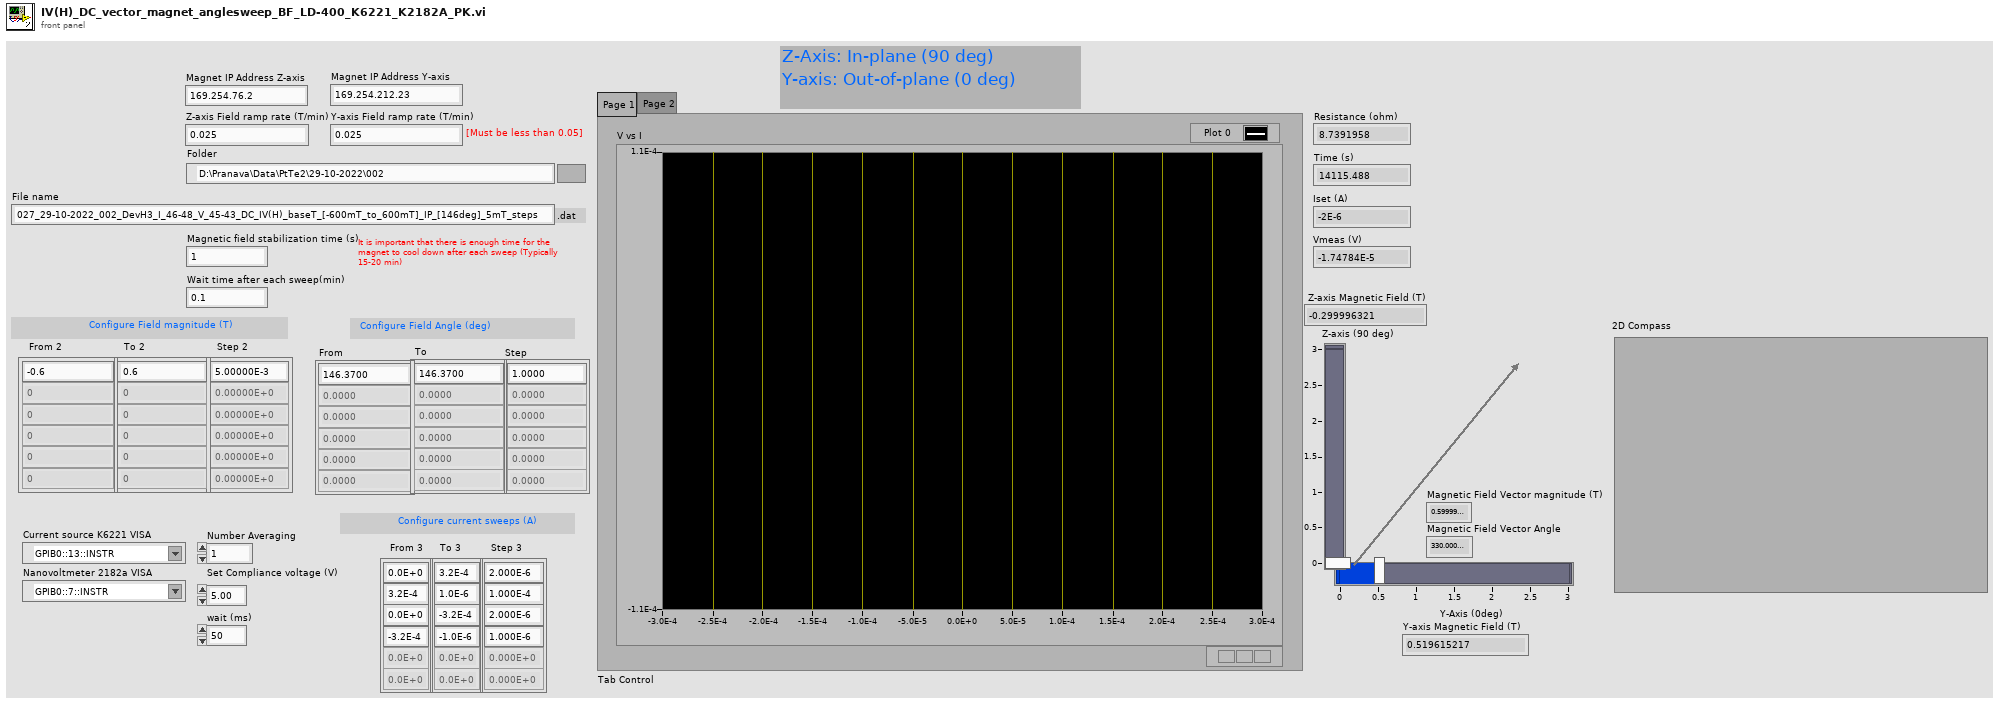
[diagram p1: front panel]
types:
  T1 = enum16{"open", "replace", "create", "open or create", "replace or create", "replace or create with confirmation"}
  T2 = typedef "Keithley 622x.lvlib/KE622x -- Current Level.ctl" = dbl
  T3 = cluster{"Average value":dbl, "Average value":dbl}
  T4 = cluster{"Average value":dbl, "Average value":dbl}[]
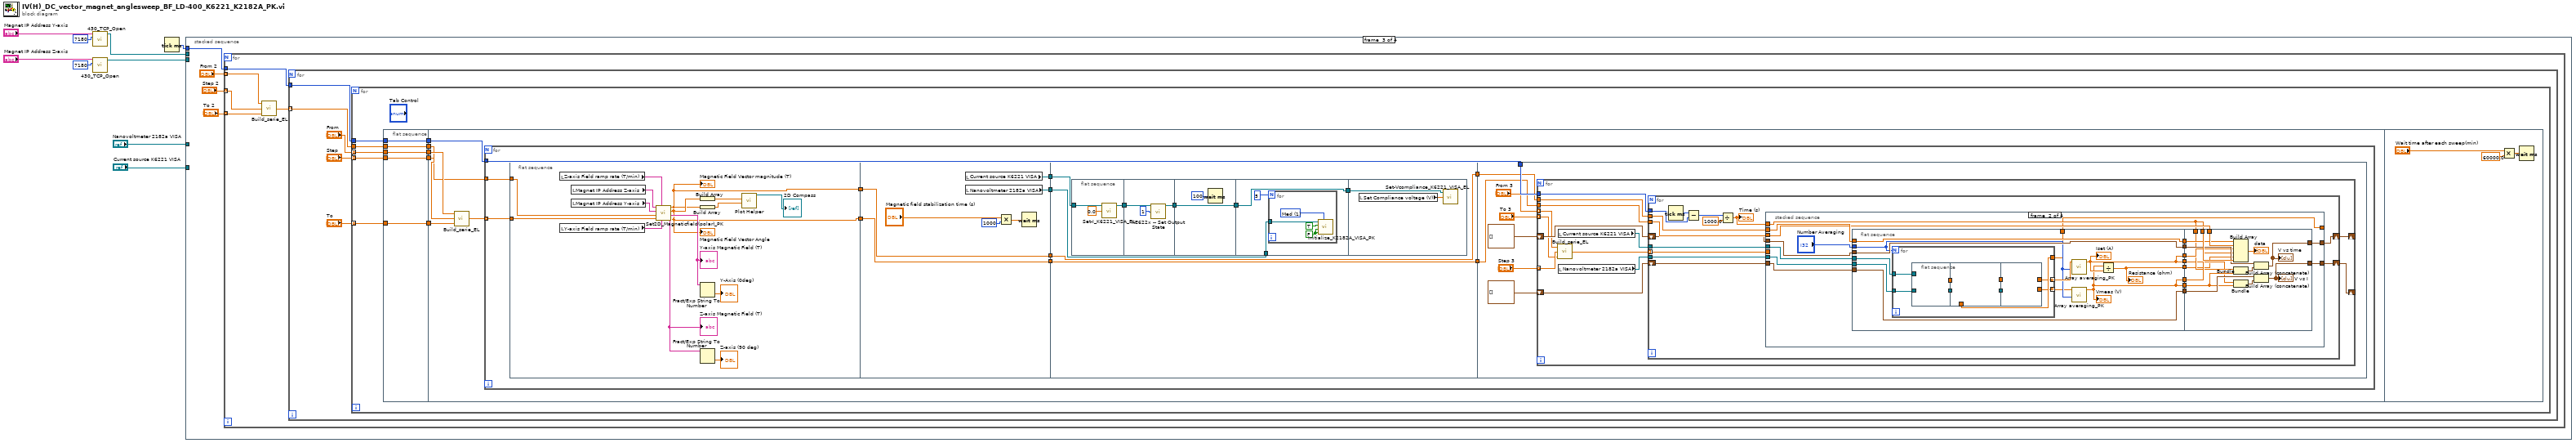
[diagram p0: block diagram]
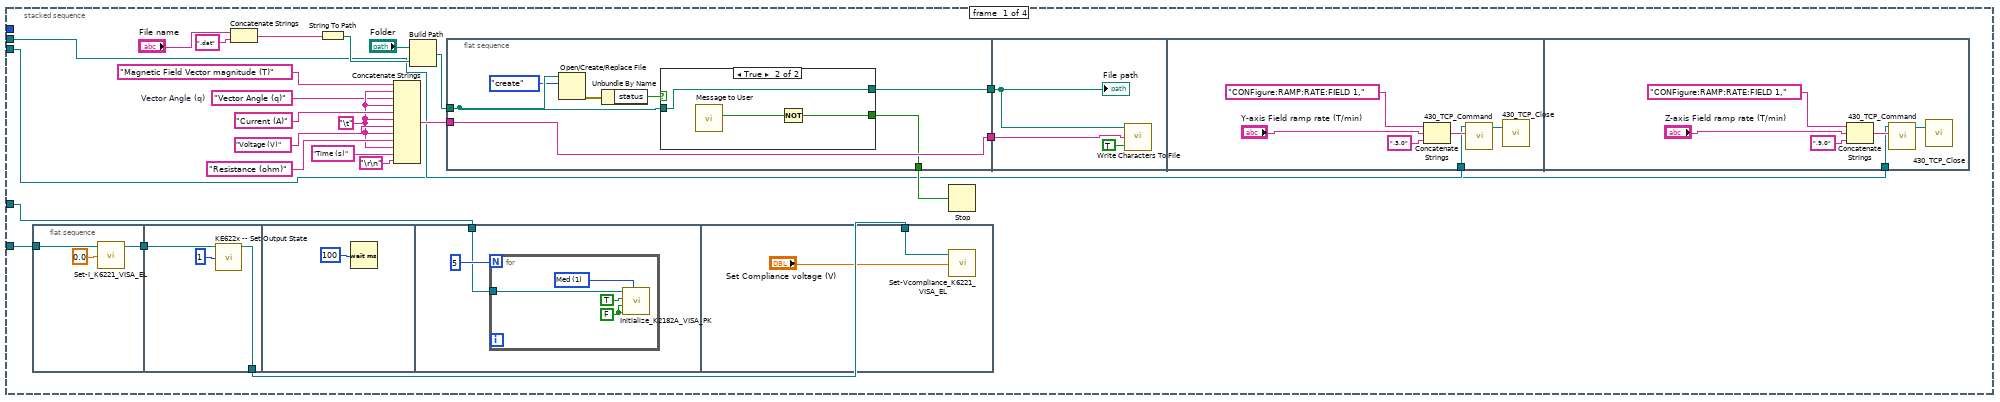
[diagram p2: hidden frame]
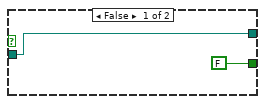
[diagram p3: hidden frame]
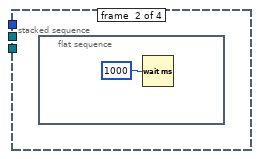
[diagram p4: hidden frame]
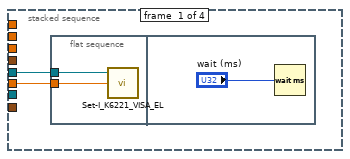
[diagram p5: hidden frame]
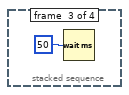
[diagram p6: hidden frame]
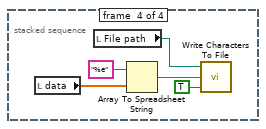
[diagram p7: hidden frame]
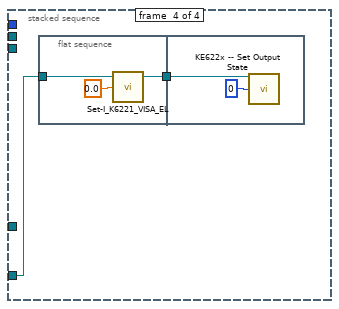
[diagram p8: hidden frame]
diagram:
  n1 = call "430_TCP_Open.vi"("IP Address"="Magnet IP Address Y-axis", "TCP Port"=7180) -> ("connection ID"=w8:refnum<k5>)  [unwired: 4 in, 2 out]
  n2 = call "430_TCP_Open.vi"("IP Address"="Magnet IP Address Z-axis", "TCP Port"=7180) -> ("connection ID"=w3:refnum<k5>)  [unwired: 4 in, 2 out]
  n3 = Tick Count (ms)() -> (millisecond timer value=w7:u32)
  n4 = stacked-sequence {
    tunnel: w8 -> [w19 _ _ _]
    tunnel: w7 -> [_ _ w80 _]
    tunnel: w3 -> [w16 _ _ _]
    tunnel: "Current source K6221 VISA" -> [w12 _ _ w284]
    tunnel: "Nanovoltmeter 2182a VISA" -> [w11 _ _ _]
    frame #0 {
      w14 = "Vector Angle (q)"  # Vector Angle (q)
      w15 = "\t"
      n5 = flat-sequence {
        tunnel: w12 -> [w36]
        tunnel: [w34] -> w13
        tunnel: w13 -> [w39]
        tunnel: [w37] -> w10
        tunnel: w11 -> [w41]
        tunnel: w10 -> [w47]
        frame #0 {
          n6 = call "Set-I_K6221_VISA_EL.vi"("Set I (A)"=0.0, "K6221 VISA"=w36) -> ("K6221 VISA out"=w34:refnum<visa-resource-name>)  [unwired: 2 in, 1 out]
        }
        frame #1 {
          n7 = call "KE622x -- Set Output State.vi"("Resource In"=w39, "Output State"=1) -> ("Resource Out (dupl)"=w37:refnum<visa-resource-name>)  [unwired: 12 in, 1 out]
        }
        frame #2 {
          n8 = Wait (ms)(milliseconds to wait=100) -> ()  [unwired: 1 out]
        }
        frame #3 {
          n9 = for {
            N: 5 ("Numeric") -> [_]
            tunnel: w41 -> [w43]
            w45 = u16 1 items=["Slow", "Med", "Fast"] ("Rate (NPLC)")
            w46 = FALSE ("Auto range?")
            n10 = call "Initialize_K2182A_VISA_PK.vi"("VISA address"=w43, "Auto range?"=TRUE, "Analog LPass\nFilter?"=w46, "DC\nFilter?"=w46, "Rate (NPLC)"=w45) -> ()  [unwired: 2 in]
          }
        }
        frame #4 {
          n11 = call "Set-Vcompliance_K6221_VISA_EL.vi"("Set Compliance voltage (V)"="Set Compliance voltage (V)", "K6221 VISA"=w47) -> ()  [unwired: 2 in, 2 out]
        }
      }
      n12 = Concatenate Strings("File name", ".dat" ("string")) -> (w29:string)
      n13 = String To Path(string=w29) -> (path=w21:path)
      n14 = Concatenate Strings("Magnetic Field Vector magnitude (T)", w15, w14, w15, "Current (A)" ("string"), w15, "Voltage (V)" ("string"), w15, "Resistance (ohm)" ("string"), w15, "Time (s)", "\r\n") -> (w30:string)
      n15 = Build Path(base path="Folder", name or relative path=w21) -> (appended path=w20:path)
      n16 = flat-sequence {
        tunnel: w20 -> [w52]
        tunnel: w30 -> [w55]
        tunnel: [w55] -> w33
        tunnel: [w54] -> w27
        tunnel: [w53] -> w32
        tunnel: w33 -> [w62]
        tunnel: w32 -> [w61]
        tunnel: w19 -> [w65]
        tunnel: w16 -> [w70]
        frame #0 {
          n17 = Open/Create/Replace File(file path (use dialog)=w52, operation (0:open)=T1."create") -> (error out=w51:errorcluster)  [unwired: 4 in, 2 out]
          n18 = Unbundle By Name(w51) -> ("status"=w49:bool)
          n19 = case shown="True" w49 {
            tunnel: [FALSE ("Yes") w59] -> w54
            tunnel: [w56 w58] -> w53
            tunnel: w52 -> [w56 w58]
            frame False {
            }
            frame True {
              n20 = call "Message to User"() -> ("Yes"=w60:bool)  [unwired: 10 in, 1 out]
              n21 = Not(x=w60) -> (.not. x?=w59:bool)
            }
          }
        }
        frame #1 {
          n22 = call <vilib>:"Write Characters To File.vi"("append to file? (new file:F)"=TRUE, "character string"=w62, "file path (dialog if empty)"=w61) -> ()  [unwired: 2 in, 1 out]
          "File path" <- w61
        }
        frame #2 {
          n23 = Concatenate Strings("CONFigure:RAMP:RATE:FIELD 1," ("String"), "Y-axis Field ramp rate (T/min)", ",3.0") -> (w66:string)
          n24 = call "430_TCP_Command.vi"("Command"=w66, "connection ID"=w65) -> ("connection ID out"=w69:refnum<k5>)  [unwired: 2 in, 2 out]
          n25 = call "430_TCP_Close.vi"("connection ID"=w69) -> ()  [unwired: 1 in, 2 out]
        }
        frame #3 {
          n26 = Concatenate Strings("CONFigure:RAMP:RATE:FIELD 1," ("String"), "Z-axis Field ramp rate (T/min)", ",9.0") -> (w72:string)
          n27 = call "430_TCP_Command.vi"("Command"=w72, "connection ID"=w70) -> ("connection ID out"=w75:refnum<k5>)  [unwired: 2 in, 2 out]
          n28 = call "430_TCP_Close.vi"("connection ID"=w75) -> ()  [unwired: 1 in, 2 out]
        }
      }
      n29 = Stop(stop? (T)=w27) -> ()
    }
    frame #1 {
      n30 = flat-sequence {
        frame #0 {
          n31 = Wait (ms)(milliseconds to wait=u32 1000) -> ()  [unwired: 1 out]
        }
      }
    }
    frame #2 {
      n32 = for {
        tunnel: w80 -> [w85]
        tunnel: "From 2" -> [w84] mode=indexing
        tunnel: "To 2" -> [w83] mode=indexing
        tunnel: "Step 2" -> [w82] mode=indexing
        n33 = call "Build_serie_EL.vi"("end value"=w83, "increment"=w82, "start value"=w84) -> ("output array"=w81:dbl[])
        n34 = for {
          tunnel: w85 -> [w87]
          tunnel: w81 -> [w86] mode=indexing
          n35 = for {
            tunnel: "From" -> [w100] mode=indexing
            tunnel: "To" -> [w98] mode=indexing
            tunnel: "Step" -> [w99] mode=indexing
            tunnel: w87 -> [w97]
            tunnel: w86 -> [w92]
            n36 = flat-sequence {
              tunnel: w97 -> [w102]
              tunnel: w98 -> [w103]
              tunnel: w99 -> [w104]
              tunnel: w100 -> [w105]
              tunnel: [w105] -> w96
              tunnel: [w104] -> w95
              tunnel: [w103] -> w94
              tunnel: [w102] -> w93
              tunnel: w92 -> [w101]
              tunnel: [w101] -> w91
              tunnel: w96 -> [w111]
              tunnel: w95 -> [w110]
              tunnel: w94 -> [w109]
              tunnel: w93 -> [w107]
              tunnel: w91 -> [w106]
              frame #0 {
              }
              frame #1 {
                n37 = call "Build_serie_EL.vi"("end value"=w109, "increment"=w110, "start value"=w111) -> ("output array"=w108:dbl[])
                n38 = for {
                  tunnel: w108 -> [w122] mode=indexing
                  tunnel: w107 -> [w121]
                  tunnel: w106 -> [w120]
                  n39 = flat-sequence {
                    tunnel: [w125] -> w119
                    tunnel: [w126] -> w118
                    tunnel: w120 -> [w123]
                    tunnel: w122 -> [w124]
                    tunnel: w119 -> [w141]
                    tunnel: [w141] -> w115
                    tunnel: [w140] -> w117
                    tunnel: w118 -> [w140]
                    tunnel: [w139] -> w113
                    tunnel: [w138] -> w112
                    tunnel: w117 -> [w152]
                    tunnel: [w152] -> w116
                    tunnel: w115 -> [w151]
                    tunnel: [w151] -> w114
                    tunnel: w113 -> [w146]
                    tunnel: w112 -> [w145]
                    tunnel: w116 -> [w175]
                    tunnel: w114 -> [w176]
                    tunnel: w121 -> [w177]
                    frame #0 {
                      n40 = local read "Z-axis Field ramp rate (T/min)"() -> (w134:string)
                      n41 = local read "Y-axis Field ramp rate (T/min)"() -> (w135:string)
                      n42 = local read "Magnet IP Address Z-axis"() -> (w137:string)
                      n43 = local read "Magnet IP Address Y-axis"() -> (w136:string)
                      n44 = call "Set2D_Magneticfield(polar)_PK.vi"("Y-axis Ramp Rate (T/min)"=w135, "Z-axis Ramp Rate (T/min)"=w134, "Set target vector angle (degrees)"=w124, "Set target vector magnitude (T)"=w123, "Y-Axis Magnet IP Address"=w136, "Z-Axis Magnet IP Address"=w137) -> ("Z-axis Magnetic Field (T)"=w131:string, "Y-axis Magnetic Field (T)"=w133:string, "q - Vector angle"=w126:dbl, "R - Vector field magnitude (T)"=w125:dbl)  [unwired: 2 in]
                      "Z-axis Magnetic Field (T)" <- w131
                      "Y-axis Magnetic Field (T)" <- w133
                      "Magnetic Field Vector magnitude (T)" <- w125
                      "Magnetic Field Vector Angle" <- w126
                      n45 = Build Array(w126) -> (w127:dbl[])
                      n46 = Build Array(w125) -> (w128:dbl[])
                      n47 = Fract/Exp String To Number(string=w133) -> (number=→"Y-Axis (0deg)":dbl)  [unwired: 3 in, 1 out]
                      n48 = Fract/Exp String To Number(string=w131) -> (number=→"Z-axis (90 deg)":dbl)  [unwired: 3 in, 1 out]
                      n49 = call-poly <vilib>:"Plot Helper.vi"("radius vector"=w128, "theta vector"=w127) -> ("2D Plot Class Obj Array out"=→"2D Compass":refnum<class "2D Plot Datatype.lvclass">[])  [unwired: 2 in, 7 out]
                    }
                    frame #1 {
                      n50 = local read "Current source K6221 VISA"() -> (w139:refnum<visa-resource-name>)
                      n51 = local read "Nanovoltmeter 2182a VISA"() -> (w138:refnum<visa-resource-name>)
                      n52 = Multiply(x="Magnetic field stabilization time (s)", y=1000) -> (x*y=w143:dbl)
                      n53 = Wait (ms)(milliseconds to wait=w143) -> ()  [unwired: 1 out]
                    }
                    frame #2 {
                      n54 = flat-sequence {
                        tunnel: w146 -> [w155]
                        tunnel: [w153] -> w150
                        tunnel: w150 -> [w158]
                        tunnel: [w156] -> w149
                        tunnel: w149 -> [w159]
                        tunnel: [w159] -> w148
                        tunnel: w148 -> [w162]
                        tunnel: [w162] -> w147
                        tunnel: w145 -> [w161]
                        tunnel: w147 -> [w168]
                        frame #0 {
                          n55 = call "Set-I_K6221_VISA_EL.vi"("Set I (A)"=0.0, "K6221 VISA"=w155) -> ("K6221 VISA out"=w153:refnum<visa-resource-name>)  [unwired: 2 in, 1 out]
                        }
                        frame #1 {
                          n56 = call "KE622x -- Set Output State.vi"("Resource In"=w158, "Output State"=1) -> ("Resource Out (dupl)"=w156:refnum<visa-resource-name>)  [unwired: 12 in, 1 out]
                        }
                        frame #2 {
                          n57 = Wait (ms)(milliseconds to wait=100) -> ()  [unwired: 1 out]
                        }
                        frame #3 {
                          n58 = for {
                            N: 5 ("Numeric") -> [_]
                            tunnel: w161 -> [w164]
                            w166 = u16 1 items=["Slow", "Med", "Fast"] ("Rate (NPLC)")
                            w167 = FALSE ("Auto range?")
                            n59 = call "Initialize_K2182A_VISA_PK.vi"("VISA address"=w164, "Auto range?"=TRUE, "Analog LPass\nFilter?"=w167, "DC\nFilter?"=w167, "Rate (NPLC)"=w166) -> ()  [unwired: 2 in]
                          }
                        }
                        frame #4 {
                          n60 = local read "Set Compliance voltage (V)"() -> (w169:dbl)
                          n61 = call "Set-Vcompliance_K6221_VISA_EL.vi"("Set Compliance voltage (V)"=w169, "K6221 VISA"=w168) -> ()  [unwired: 2 in, 2 out]
                        }
                      }
                    }
                    frame #3 {
                      n62 = for {
                        tunnel: w177 -> [w190]
                        tunnel: w176 -> [w188]
                        tunnel: w175 -> [w187]
                        tunnel: "From 3" -> [w182] mode=indexing
                        tunnel: "Step 3" -> [w181] mode=indexing
                        tunnel: "To 3" -> [w180] mode=indexing
                        shift-right: [w179] -> _
                        shift-left: cluster{dbl, "Field Reading":dbl}[] [] -> [w186]
                        shift-right: [w178] -> _
                        shift-left: cluster{dbl, "Field Reading":dbl}[] [] -> [w189]
                        n63 = call "Build_serie_EL.vi"("end value"=w180, "increment"=w181, "start value"=w182) -> ("output array"=w183:dbl[])
                        n64 = local read "Current source K6221 VISA"() -> (w185:refnum<visa-resource-name>)
                        n65 = local read "Nanovoltmeter 2182a VISA"() -> (w184:refnum<visa-resource-name>)
                        n66 = for {
                          tunnel: w190 -> [w204]
                          tunnel: w188 -> [w198]
                          tunnel: w187 -> [w197]
                          tunnel: w183 -> [w195] mode=indexing
                          shift-right: [w191] -> w178
                          shift-left: w189 -> [w203]
                          shift-right: [w192] -> w179
                          shift-left: w186 -> [w196]
                          tunnel: w185 -> [w194]
                          tunnel: w184 -> [w193]
                          n67 = Tick Count (ms)() -> (millisecond timer value=w200:u32)
                          n68 = Subtract(x=w200, y=w204) -> (x-y=w202:u32)
                          n69 = Divide(x=w202, y=1000.0) -> (x/y=w199:dbl)
                          "Time (s)" <- w199
                          n70 = stacked-sequence {
                            tunnel: w203 -> [_ w227 _ _]
                            tunnel: [_ w228 _ _] -> w191
                            tunnel: w199 -> [_ w215 _ _]
                            tunnel: w198 -> [_ w222 _ _]
                            tunnel: w197 -> [_ w221 _ _]
                            tunnel: [_ w220 _ _] -> w192
                            tunnel: w196 -> [_ w218 _ _]
                            tunnel: w195 -> [w206 _ _ _]
                            tunnel: [_ w212 _ _] -> _
                            tunnel: w194 -> [w205 w211 _ _]
                            tunnel: w193 -> [_ w210 _ _]
                            frame #0 {
                              n71 = flat-sequence {
                                tunnel: w206 -> [w208]
                                tunnel: w205 -> [w207]
                                frame #0 {
                                n72 = call "Set-I_K6221_VISA_EL.vi"("Set I (A)"=w208, "K6221 VISA"=w207) -> ()  [unwired: 2 in, 2 out]
                                }
                                frame #1 {
                                n73 = Wait (ms)(milliseconds to wait="wait (ms)") -> ()  [unwired: 1 out]
                                }
                              }
                            }
                            frame #1 {
                              n74 = flat-sequence {
                                tunnel: [w234] -> w226
                                tunnel: [w240] -> w225
                                tunnel: [w236] -> w224
                                tunnel: [w239] -> w223
                                tunnel: [w238] -> w219
                                tunnel: "Number Averaging" -> [w233]
                                tunnel: w218 -> [w238]
                                tunnel: w227 -> [w240]
                                tunnel: w222 -> [w239]
                                tunnel: [w234] -> w216
                                tunnel: [w236] -> w214
                                tunnel: [w237] -> w213
                                tunnel: [w231] -> w212
                                tunnel: w211 -> [w230]
                                tunnel: w210 -> [w229]
                                tunnel: w226 -> [w263]
                                tunnel: [w273] -> w228
                                tunnel: w225 -> [w272]
                                tunnel: w224 -> [w262]
                                tunnel: w223 -> [w267]
                                tunnel: w215 -> [w270]
                                tunnel: w221 -> [w269]
                                tunnel: [w265] -> w220
                                tunnel: w219 -> [w264]
                                tunnel: w216 -> [w266]
                                tunnel: w215 -> [w261]
                                tunnel: w214 -> [w260]
                                tunnel: w213 -> [w259]
                                frame #0 {
                                n75 = for {
                                N: w233 -> [_]
                                tunnel: [w242] -> w232 mode=indexing
                                tunnel: [w241] -> w235 mode=indexing
                                tunnel: w230 -> [w248]
                                tunnel: [w247] -> w231
                                tunnel: w229 -> [w249]
                                n76 = flat-sequence {
                                tunnel: w248 -> [w250]
                                tunnel: w249 -> [w252]
                                tunnel: [w252] -> w246
                                tunnel: [w251] -> w245
                                tunnel: [w254] -> w247
                                tunnel: w246 -> [w255]
                                tunnel: w245 -> [w254]
                                tunnel: [w255] -> w244
                                tunnel: [w254] -> w243
                                tunnel: [w258] -> w241
                                tunnel: w244 -> [w257]
                                tunnel: w243 -> [w258]
                                tunnel: [w256] -> w242
                                frame #0 {
                                n77 = call "KE622x -- Get Current Level.vi"("Resource In"=w250) -> ("Current Level (A)"=w251:T2)  [unwired: 12 in, 2 out]
                                }
                                frame #1 {
                                n78 = Wait (ms)(milliseconds to wait=50) -> ()  [unwired: 1 out]
                                }
                                frame #2 {
                                n79 = call "Get-V_K2182A_VISA_EL.vi"("VISA K2182A"=w257) -> ("V (V)"=w256:dbl)  [unwired: 2 in, 2 out]
                                }
                                }
                                }
                                n80 = call "Array averaging_PK.vi"("Number averaging"=w233, "numeric array"=w235) -> ("Average value"=w236:dbl)  [unwired: 9 in]
                                "Iset (A)" <- w236
                                n81 = call "Array averaging_PK.vi"("Number averaging"=w233, "numeric array"=w232) -> ("Average value"=w234:dbl)  [unwired: 9 in]
                                "Vmeas (V)" <- w234
                                n82 = Divide(x=w234, y=w236) -> (x/y=w237:dbl)
                                "Resistance (ohm)" <- w237
                                }
                                frame #1 {
                                n83 = Build Array(w267, w269, w262, w263, w259, w270) -> (→"data":dbl[])
                                n84 = Bundle(w261, "Average value"=w266) -> (w268:cluster{dbl, "Average value":dbl})  [unwired: 1 in]
                                n85 = Bundle("Average value"=w260, "Average value"=w266) -> (w271:T3)  [unwired: 1 in]
                                n86 = Build Array (concatenate)(w264, w268) -> (w265:cluster{dbl, "Average value":dbl}[])
                                "V vs time" <- w265
                                n87 = Build Array (concatenate)(w272, w271) -> (w273:T4)
                                "V vs I" <- w273
                                }
                              }
                            }
                            frame #2 {
                              n88 = Wait (ms)(milliseconds to wait=u32 50) -> ()  [unwired: 1 out]
                            }
                            frame #3 {
                              n89 = local read "data"() -> (w276:dbl[])
                              n90 = local read "File path"() -> (w278:path)
                              n91 = Array To Spreadsheet String(array=w276, 3:"%e" ("format string")) -> (spreadsheet string=w279:string)  [unwired: 1 in]
                              n92 = call <vilib>:"Write Characters To File.vi"("append to file? (new file:F)"=TRUE, "character string"=w279, "file path (dialog if empty)"=w278) -> ()  [unwired: 2 in, 1 out]
                            }
                          }
                        }
                      }
                    }
                  }
                }
              }
              frame #2 {
                n93 = Multiply(x="Wait time after each sweep(min)", y=60000.0) -> (x*y=w283:dbl)
                n94 = Wait (ms)(milliseconds to wait=w283) -> ()  [unwired: 1 out]
              }
            }
          }
        }
      }
    }
    frame #3 {
      n95 = flat-sequence {
        tunnel: w284 -> [w288]
        tunnel: [w286] -> w285
        tunnel: w285 -> [w290]
        frame #0 {
          n96 = call "Set-I_K6221_VISA_EL.vi"("Set I (A)"=0.0, "K6221 VISA"=w288) -> ("K6221 VISA out"=w286:refnum<visa-resource-name>)  [unwired: 2 in, 1 out]
        }
        frame #1 {
          n97 = call "KE622x -- Set Output State.vi"("Resource In"=w290, "Output State"=0) -> ()  [unwired: 12 in, 2 out]
        }
      }
    }
  }
